vi "图片居中.vi"(6 "原始图片尺寸":T1={"left"=0, "top"=0, "right"=1262, "bottom"=948}, 7 "背景色（黑）":picture, 8 "错误输入（无错误）":errorcluster, 11 "图片引用":refnum<vi>) -> (0 "错误输出":errorcluster, 4 "Rectangle":T1)   [LabVIEW 2016]
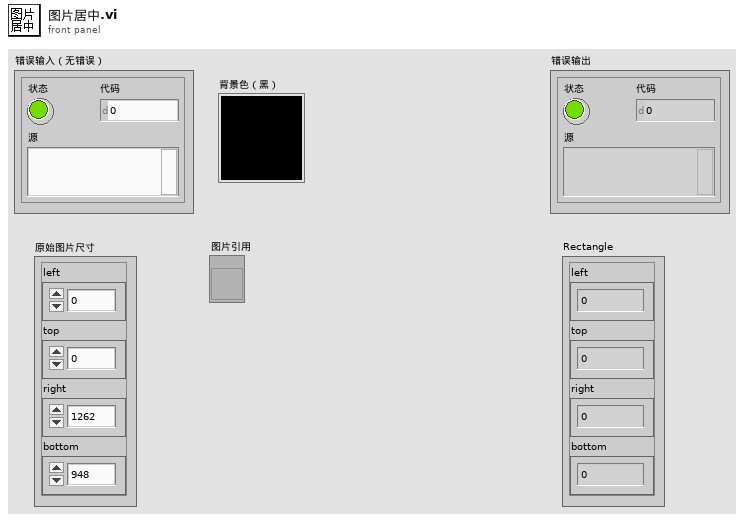
[diagram p1: front panel]
types:
  T1 = cluster{"left":i16, "top":i16, "right":i16, "bottom":i16}
  T2 = typedef "LVBoundsTypeDef.ctl" = cluster{"Width":u32, "Height":u32}
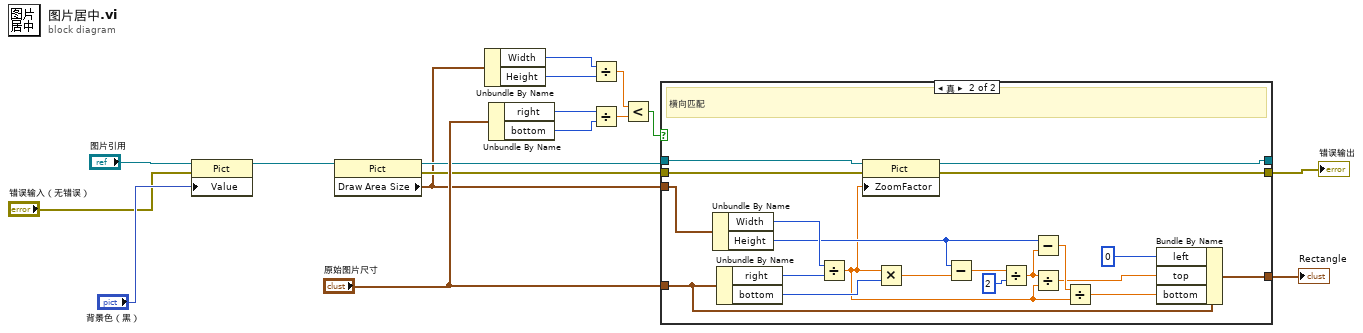
[diagram p0: block diagram]
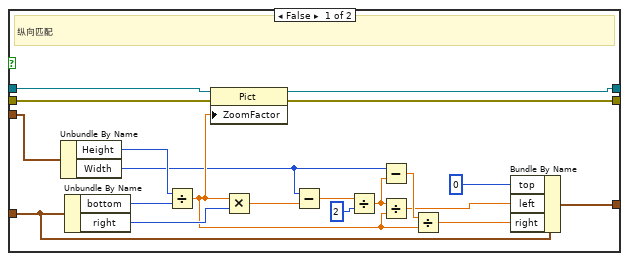
[diagram p2: hidden frame]
diagram:
  n1 = property class="Pict"(reference="图片引用", error in="错误输入（无错误）", "Value"="背景色（黑）") -> (reference out=w16:refnum<vi>)  [unwired: 1 out]
  n2 = property on="属性节点" class="Pict"(reference=w16) -> (reference out=w12:refnum<vi>, error out=w13:errorcluster, "Draw Area Size"=w11:T2)  [unwired: 1 in]
  n3 = Unbundle By Name(w11) -> ("Width"=w8:u32, "Height"=w9:u32)
  n4 = Unbundle By Name("原始图片尺寸") -> ("right"=w15:i16, "bottom"=w10:i16)
  n5 = Divide(x=w8, y=w9) -> (x/y=w5:dbl)
  n6 = Divide(x=w15, y=w10) -> (x/y=w6:dbl)
  n7 = Less?(x=w5, y=w6) -> (x < y?=w7:bool)
  n8 = case shown="真" w7 {
    tunnel: w11 -> [w37 w57]
    tunnel: "原始图片尺寸" -> [w28 w48]
    tunnel: [w32 w52] -> w3
    tunnel: w12 -> [w21 w41]
    tunnel: w13 -> [w20 w40]
    tunnel: [w19 w39] -> w1
    tunnel: [w18 w38] -> _
    frame False {
      # "纵向匹配"
      n9 = Unbundle By Name(w37) -> ("Height"=w36:u32, "Width"=w22:u32)
      n10 = Unbundle By Name(w28) -> ("bottom"=w31:i16, "right"=w30:i16)
      n11 = Divide(x=w36, y=w31) -> (x/y=w24:dbl)
      n12 = property on="属性节点" class="Pict"(reference=w21, error in=w20, "ZoomFactor"=w24) -> (reference out=w18:refnum<vi>, error out=w19:errorcluster)
      n13 = Multiply(x=w24, y=w30) -> (x*y=w29:dbl)
      n14 = Subtract(x=w22, y=w29) -> (x-y=w34:dbl)
      n15 = Divide(x=w34, y=u32 2) -> (x/y=w23:dbl)
      n16 = Subtract(x=w22, y=w23) -> (x-y=w27:dbl)
      n17 = Divide(x=w23, y=w24) -> (x/y=w26:dbl)
      n18 = Divide(x=w27, y=w24) -> (x/y=w25:dbl)
      n19 = Bundle By Name(cluster=w28, "top"=i16 0 ("Rectangle.left"), "left"=w26, "right"=w25) -> (w32:T1)
    }
    frame True {
      # "横向匹配"
      n20 = Unbundle By Name(w57) -> ("Width"=w56:u32, "Height"=w47:u32)
      n21 = Unbundle By Name(w48) -> ("right"=w51:i16, "bottom"=w50:i16)
      n22 = Divide(x=w56, y=w51) -> (x/y=w42:dbl)
      n23 = property on="属性节点" class="Pict"(reference=w41, error in=w40, "ZoomFactor"=w42) -> (reference out=w38:refnum<vi>, error out=w39:errorcluster)
      n24 = Multiply(x=w42, y=w50) -> (x*y=w49:dbl)
      n25 = Subtract(x=w47, y=w49) -> (x-y=w54:dbl)
      n26 = Divide(x=w54, y=u32 2) -> (x/y=w45:dbl)
      n27 = Subtract(x=w47, y=w45) -> (x-y=w46:dbl)
      n28 = Divide(x=w45, y=w42) -> (x/y=w44:dbl)
      n29 = Divide(x=w46, y=w42) -> (x/y=w43:dbl)
      n30 = Bundle By Name(cluster=w48, "left"=i16 0 ("Rectangle.left"), "top"=w44, "bottom"=w43) -> (w52:T1)
    }
  }
  "Rectangle" <- w3
  "错误输出" <- w1
